vi "Result._TEST CSV result file to Array of Meas.vi"(8 "error in":errorcluster, 11 "Path":path) -> (0 "error out":errorcluster, 3 "Meas":T1[](array[typedef]) {"Status" items=["LOG", "PASS", "FAIL", "ERROR"]})   [LabVIEW 2019]
uses:
  Result.Measurement Item.ctl
  Result.Measurement and Attribute Item Status.ctl
  Errors/Error.Error Code List.ctl
  <vilib>/KATE/Files/File Utils.lvlib
  <vilib>/KATE/Strings/String Utils.lvlib
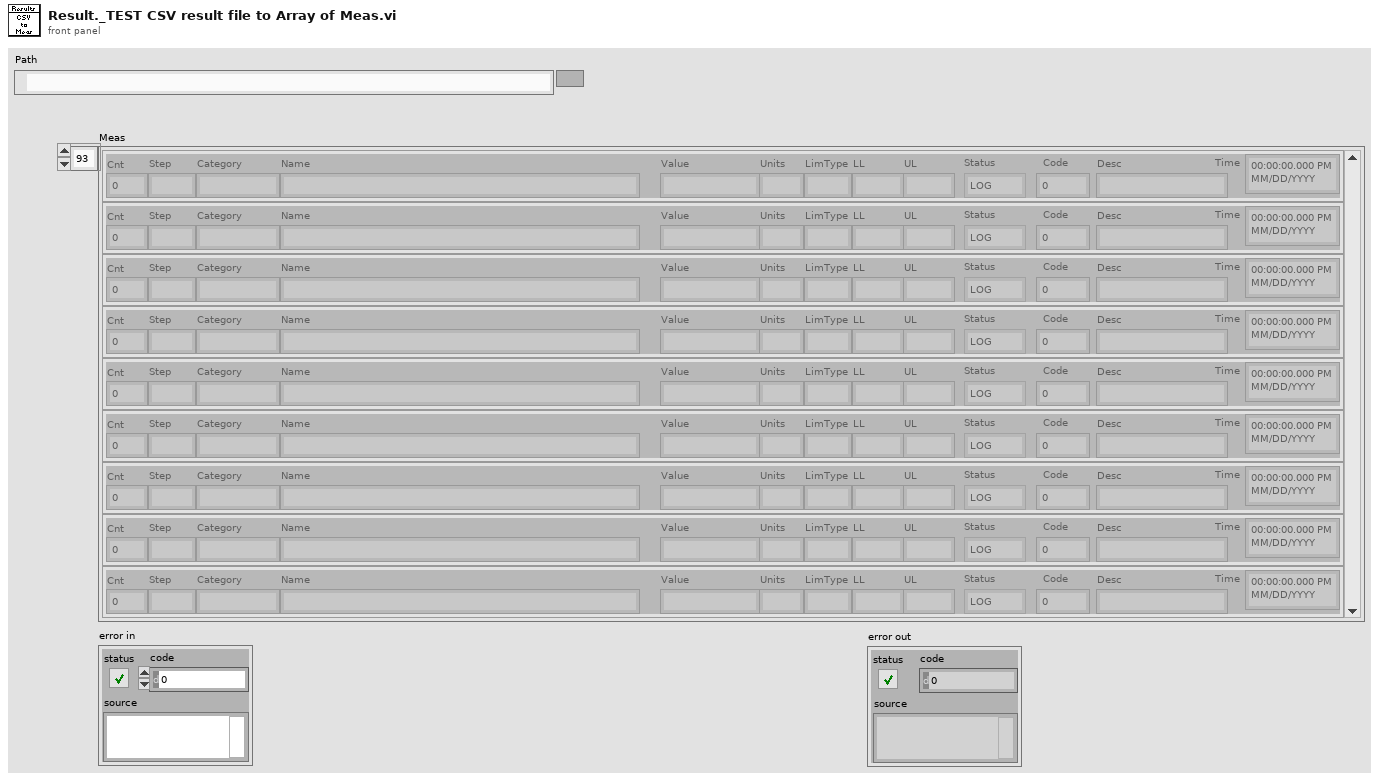
[diagram p1: front panel]
types:
  T1 = typedef "Result.Measurement Item.ctl" = cluster{"Cnt":i32, "Step":string, "Category":string, "Name":string, "Value":string, "Units":string, "LimType":string, "LL":string, "UL":string, "Status":T2, "Code":i32, "Desc":string, "Time":timestamp}
  T2 = typedef "Result.Measurement and Attribute Item Status.ctl" = i32
  T3 = typedef "Error.Error Code List.ctl" = i32
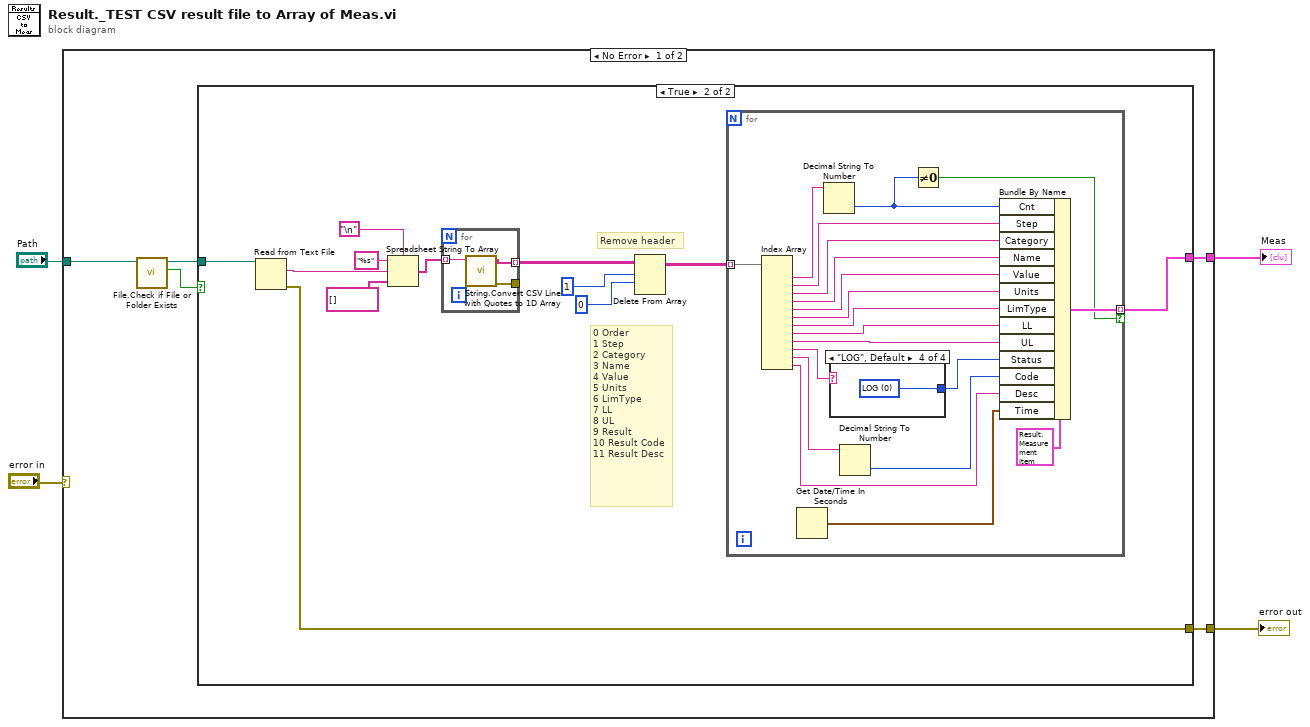
[diagram p0: block diagram]
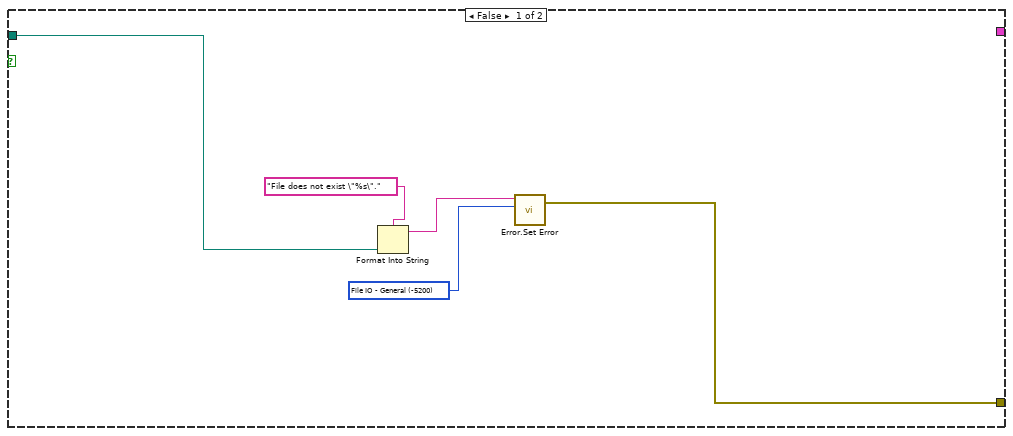
[diagram p2: hidden frame]
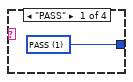
[diagram p3: hidden frame]
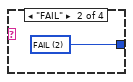
[diagram p4: hidden frame]
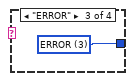
[diagram p5: hidden frame]
diagram:
  n1 = case shown="No Error" "error in" {
    selector: "error in" -> [_ w54]
    tunnel: "Path" -> [w9 _]
    tunnel: [w6 w54] -> w2
    tunnel: [w5 _] -> w1
    frame No Error {
      n2 = call <vilib>:"File.Check if File or Folder Exists.vi"("Path"=w9) -> ("Exists"=w8:bool, "Dup Path"=w7:path)  [unwired: 6 in, 3 out]
      n3 = case shown="True" w8 {
        tunnel: w7 -> [w13 w26]
        tunnel: [w10 w17] -> w6
        tunnel: [_ w15] -> w5
        frame False {
          w11 = T3 -5200 items=["No Error"=0, "Abort"=-2, "Misc"=-5000, "Fixture Error"=-5100, "File IO - General"=-5200, "FIle IO - Config Error"=-5201, "Instrument - General"=-5300, "Instrument - Serial Com"=-5301, "Instrument - Camera"=-5302, "Instrument - PS"=-5303, "Instrument - Oscilloscope"=-5304, "Instrument - Function Gen"=-5305, "Instrument - Load"=-5306, "Instrument - Meter"=-5307, "Instrument - Power Control"=-5308, "Instrument - Motion"=-5309, "Instrument - RF"=-5310, "System Exe"=-5400, "Image Processing"=-5500, "Communication"=-5600, "Script - Syntax Error"=-6000, "Script - Invalid Name or Param"=-6100, "Script - Timeout"=-6200, "Invalid Data"=-6300, "FW Update Error"=-6500] ("Std Code")
          n4 = Format Into String(format string="File does not exist \"%s\".", w13) -> (resulting string=w12:string)  [unwired: 2 in, 1 out]
          n5 = call "Error.Set Error.vi"("Code"=w11, "Desc"=w12) -> ("error out"=w10:errorcluster)  [unwired: 5 in]
        }
        frame True {
          # "0\tOrder\n1\tStep\n2\tCategory\n3\tName\n4\tValue\n5\tUnits\n6\tLimType\n7\tLL\n8\tUL\n9\tResult\n10\tResult Code\n11\tResult Desc"
          # "Remove header"
          n6 = Read from Text File(file (use dialog)=w26) -> (text=w18:string, error out=w17:errorcluster)  [unwired: 3 in, 2 out]
          n7 = Spreadsheet String To Array(delimiter (Tab)="\n", format string="%s", spreadsheet string=w18, array type (2D Dbl)=string[] [] ("Raw Data")) -> (array=w20:string[])
          n8 = for {
            tunnel: w20 -> [w53] mode=indexing
            tunnel: [w52] -> w19 mode=indexing
            tunnel: [w51] -> _
            n9 = call <vilib>:"String.Convert CSV Line with Quotes to 1D Array.vi"("CSV String"=w53) -> ("error out"=w51:errorcluster, "Array"=w52:string[])  [unwired: 9 in]
          }
          n10 = Delete From Array(array=w19, length=1, index (row)=0) -> (array with subset deleted=w16:string[][])  [unwired: 1 in, 1 out]
          n11 = for {
            tunnel: w16 -> [w46] mode=indexing
            tunnel: [w44] -> w15 mode=indexing if=w27
            n12 = Index Array(array=w46) -> (element #1=w42:string, element #2=w41:string, element #3=w40:string, element #4=w39:string, element #5=w38:string, element #6=w37:string, element #7=w36:string, element #8=w35:string, element #9=w34:string, element #10=w30:string, element #11=w33:string, element #12=w31:string)  [unwired: 12 in]
            n13 = Get Date/Time In Seconds() -> (seconds since 1Jan1904=w43:timestamp)
            n14 = Decimal String To Number(string=w42) -> (number=w28:i32)  [unwired: 2 in, 1 out]
            n15 = case shown="\"LOG\", Default" w30 {
              tunnel: [w47 w48 w49 w50] -> w29
              frame "PASS" {
                w47 = T2 1 items=["LOG", "PASS", "FAIL", "ERROR"] ("Status")
              }
              frame "FAIL" {
                w48 = T2 2 items=["LOG", "PASS", "FAIL", "ERROR"] ("Status")
              }
              frame "ERROR" {
                w49 = T2 3 items=["LOG", "PASS", "FAIL", "ERROR"] ("Status")
              }
              frame "LOG", Default {
                w50 = T2 0 items=["LOG", "PASS", "FAIL", "ERROR"] ("Status")
              }
            }
            n16 = Decimal String To Number(string=w33) -> (number=w32:i32)  [unwired: 2 in, 1 out]
            n17 = Not Equal To 0?(x=w28) -> (x != 0?=w27:bool)
            n18 = Bundle By Name(cluster=T1 {"Cnt"=0, "Step"="", "Category"="", "Name"="", "Value"="", "Units"="", "LimType"="", "LL"="", "UL"="", "Status"=0, "Code"=0, "Desc"="", "Time"=timestamp(0 s since 1904-01-01)} ("Meas"), "Cnt"=w28, "Step"=w41, "Category"=w40, "Name"=w39, "Value"=w38, "Units"=w37, "LimType"=w36, "LL"=w35, "UL"=w34, "Status"=w29, "Code"=w32, "Desc"=w31, "Time"=w43) -> (w44:T1)
          }
        }
      }
    }
    frame Error {
    }
  }
  "Meas" <- w1
  "error out" <- w2
